vi "Configure Tx.vi"(0 "niUsrpRio Session":T1={"FPGA Interface"=refnum, "RIO Interface Number"=0, "Data Clock Rate"=0, "FPGA Data Clock Rate"=0, "Global Settings Register Bus"=refnum, "Radio 0 Settings Register Bus"=refnum, "Radio 1 Settings Register Bus"=refnum, "Radio Settings Bus Semaphore"=refnum, "DB Queues"=[], "Characterization Data Valid?"=FALSE, "EEPROM Header"={"Checksum"=0, "Product Code"=0, "Hardware Current Version"=0, "Hardware Oldest Compatible Version"=0, "EEPROM Map Current Version"=0, "EEPROM Map Oldest Compatible Version"=0, "User Password"="", "Pointer to Factory Header"=0, "Pointer to User Header"=0, "Recommended Interval"=0, "Number of Reserved Bytes"=9, "Number of Daughterboards"=0, "Daughterboard IDs"=[], "Daughterboard Serial Numbers"=[]}, "Device Data Header"={"Checksum"=0, "Number of Channels"=0, "Number of Gain Settings"=[], "Pointer to Characterization Data"=[], "Number of Reserved Bytes"=27, "Number of Frequencies"=[]}, "EEPROM Characterization Header"={"Checksum"=0, "Date"=timestamp(0 s since 1904-01-01), "Temperature"=0.0, "Misc. Info"="", "Pointer to Device Data Header"=0, "Number of Reserved Bytes"=28}, "Characterization Data"=[], "FPGA Current Version"=0, "FPGA Oldest Compatible Version"=0, "Fixed Logic Current Version"=0, "Fixed Logic Oldest Compatible Version"=0, "FPGA Radio Settings Bus Current Version"=0, "FPGA Radio Settings Bus Oldest Compatible Version"=0, "FPGA Board Config Current Version"=0, "FPGA Board Config Oldest Compatible Version"=0} {"FPGA Data Clock Rate" format="%#.3pHz"; "Data Clock Rate" format="%#.3pHz"; "Characterization Data"."Frequencies [Hz]" format="%#_6p"; "EEPROM Characterization Header"."Pointer to Device Data Header" format="%x"; "EEPROM Characterization Header"."Checksum" format="%x"; "Device Data Header"."Pointer to Characterization Data" format="%x"; "Device Data Header"."Checksum" format="%x"; "EEPROM Header"."Pointer to User Header" format="%x"; "EEPROM Header"."Pointer to Factory Header" format="%x"; "EEPROM Header"."Product Code" format="%x"; "EEPROM Header"."Checksum" format="%x"}, 5 "tx config":T11={"rf enable 0"=FALSE, "rf config 0"={"antenna"="TX1", "frequency"=2000000000.0, "lo frequency"=-1.0, "level"=0.0}, "rf enable 1"=FALSE, "rf config 1"={"antenna"="TX1", "frequency"=2000000000.0, "lo frequency"=-1.0, "level"=0.0}, "transfer mode"=enum."Finite", "sample rate"=10000000.0, "number of samples"=8192, "start trigger"=enum."Immediate", "tone frequency"=100000.0} {"tone frequency" format="%#.3pHz"; "sample rate" format="%#.3pS/s"; "rf config 0"."level" format="%#_gdBm"; "rf config 0"."lo frequency" format="%#.3pHz"; "rf config 0"."frequency" format="%#.3pHz"; "rf config 1"."level" format="%#_gdBm"; "rf config 1"."lo frequency" format="%#.3pHz"; "rf config 1"."frequency" format="%#.3pHz"}, 11 "error in":errorcluster, 12 "x":cdb[](array[numeric])) -> (4 "niUsrpRio Session (out)":T1 {"FPGA Data Clock Rate" format="%#.3pHz"; "Data Clock Rate" format="%#.3pHz"; "Characterization Data"."Frequencies [Hz]" format="%#_6p"; "EEPROM Characterization Header"."Pointer to Device Data Header" format="%x"; "EEPROM Characterization Header"."Checksum" format="%x"; "Device Data Header"."Pointer to Characterization Data" format="%x"; "Device Data Header"."Checksum" format="%x"; "EEPROM Header"."Pointer to User Header" format="%x"; "EEPROM Header"."Pointer to Factory Header" format="%x"; "EEPROM Header"."Product Code" format="%x"; "EEPROM Header"."Checksum" format="%x"}, 6 "tx.enabled channels":string[](array[string]), 8 "I":i16[](array[numeric]), 10 "Q":i16[](array[numeric]), 13 "tx.output waveform":waveform(dbl)[](graph), 14 "tx.coerced configurations":T12 {"coerced sample rates" format="%#.3pS/s"; "coerced levels" format="%#.3gdBm"; "coerced lo frequencies" format="%#.3pHz"; "coerced frequencies" format="%#.3pHz"}, 15 "error out":errorcluster)   [LabVIEW 2015]
uses:
  <instrlib>/niUsrpRio/Config/v1/Host/Public/niUsrpRio Session.ctl
  <instrlib>/_niInstr/Register Bus/v0/Host/Public/Register Bus Session.ctl
  <instrlib>/_niInstr/Register Bus/v0/Host/Private/Session Data.ctl
  <instrlib>/niUsrpRio/Config/v1/Host/Private/DB Queue Reference.ctl
  <instrlib>/niUsrpRio/Config/v1/Host/Private/Daughterboard Data.ctl
  <instrlib>/niUsrpRio/Config/v1/Host/Private/ATR state data.ctl
  <instrlib>/niUsrpRio/Config/v1/Host/Public/EEPROM Header.ctl
  <instrlib>/niUsrpRio/Config/v1/Host/Public/EEPROM Device Data Header.ctl
  <instrlib>/niUsrpRio/Config/v1/Host/Public/EEPROM Characterization Header.ctl
  <instrlib>/niUsrpRio/Config/v1/Host/Public/Characterization Data.ctl
  <instrlib>/niUsrpRio/Config/v1/Host/Public/IQ Imbalance.ctl
  Start Trigger.ctl
  Configure Signal (Level).vi
  PPS_Global_Var.vi
  <instrlib>/_niInstr/Register Bus/v0/Host/niInstr Register Bus v0 Host.lvlib
  <instrlib>/niUsrpRio/Config/v1/Host/niUsrpRio Config v1 Host.lvlib
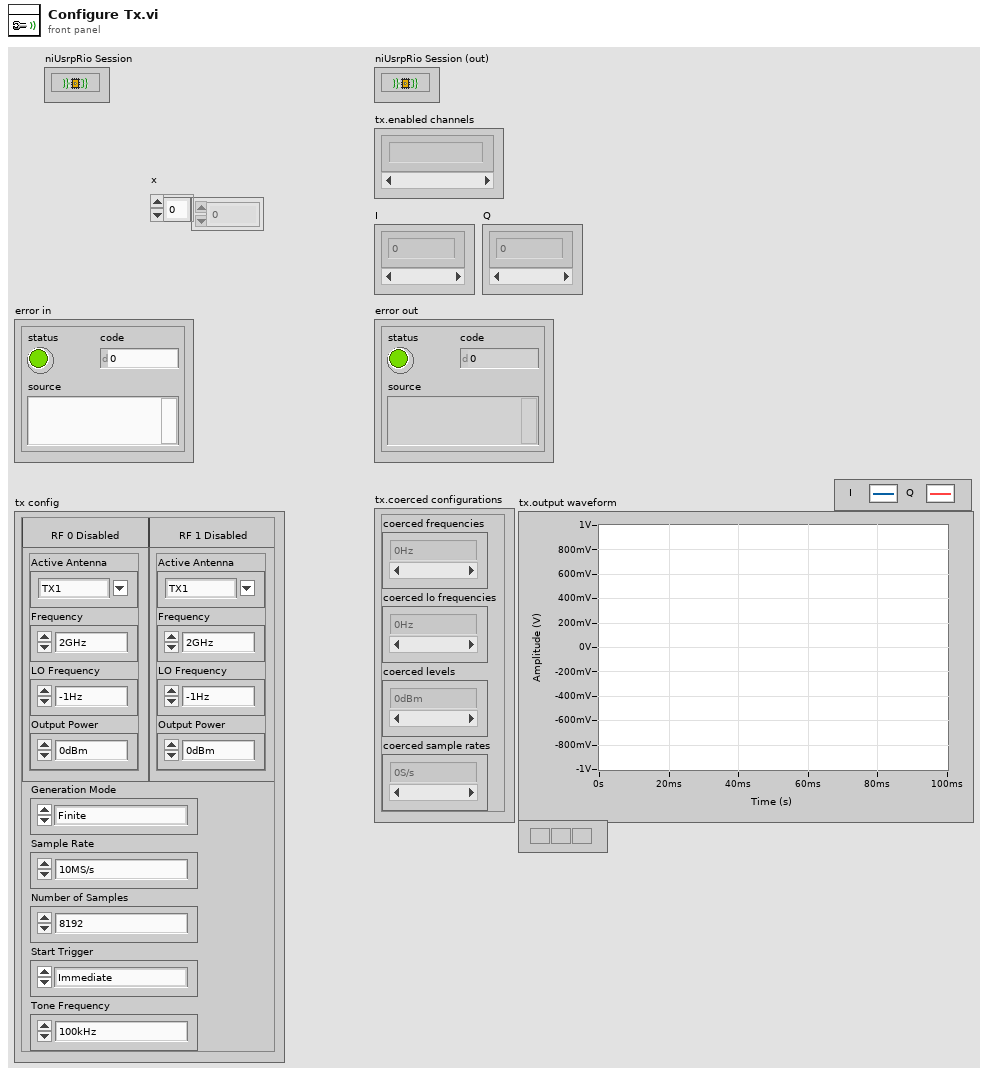
[diagram p1: front panel]
types:
  T1 = typedef "niUsrpRio Config v1 Host.lvlib/niUsrpRio Session.ctl" = cluster{"FPGA Interface":refnum<k20>, "RIO Interface Number":u32, "Data Clock Rate":u32, "FPGA Data Clock Rate":u32, "Global Settings Register Bus":T2, "Radio 0 Settings Register Bus":T2, "Radio 1 Settings Register Bus":T2, "Radio Settings Bus Semaphore":T3, "DB Queues":T4[], "Characterization Data Valid?":bool, "EEPROM Header":T5, "Device Data Header":T6, "EEPROM Characterization Header":T7, "Characterization Data":T8[], "FPGA Current Version":u32, "FPGA Oldest Compatible Version":u32, "Fixed Logic Current Version":u32, "Fixed Logic Oldest Compatible Version":u32, "FPGA Radio Settings Bus Current Version":u32, "FPGA Radio Settings Bus Oldest Compatible Version":u32, "FPGA Board Config Current Version":u32, "FPGA Board Config Oldest Compatible Version":u32}
  T2 = typedef "niInstr Register Bus v0 Host.lvlib/Register Bus Session.ctl" = refnum<queue>
  T3 = typedef "Semaphore RefNum" = refnum<k1>
  T4 = typedef "niUsrpRio Config v1 Host.lvlib/DB Queue Reference.ctl" = refnum<queue>
  T5 = typedef "niUsrpRio Config v1 Host.lvlib/EEPROM Header.ctl" = cluster{"Checksum":u32, "Product Code":u16, "Hardware Current Version":u16, "Hardware Oldest Compatible Version":u16, "EEPROM Map Current Version":u16, "EEPROM Map Oldest Compatible Version":u16, "User Password":string, "Pointer to Factory Header":u32, "Pointer to User Header":u32, "Recommended Interval":u16, "Number of Reserved Bytes":i32, "Number of Daughterboards":u8, "Daughterboard IDs":u16[], "Daughterboard Serial Numbers":string[]}
  T6 = typedef "niUsrpRio Config v1 Host.lvlib/EEPROM Device Data Header.ctl" = cluster{"Checksum":u32, "Number of Channels":u8, "Number of Gain Settings":u16[], "Pointer to Characterization Data":u32[], "Number of Reserved Bytes":i32, "Number of Frequencies":u16[]}
  T7 = typedef "niUsrpRio Config v1 Host.lvlib/EEPROM Characterization Header.ctl" = cluster{"Checksum":u32, "Date":timestamp, "Temperature":sgl, "Misc. Info":string, "Pointer to Device Data Header":u32, "Number of Reserved Bytes":i32}
  T8 = typedef "niUsrpRio Config v1 Host.lvlib/Characterization Data.ctl" = cluster{"Gains[dB]":dbl[], "Frequencies [Hz]":dbl[], "IQ Imbalance Table":T9[], "Measured Gains[dB]":dbl[][]}
  T9 = typedef "niUsrpRio Config v1 Host.lvlib/IQ Imbalance.ctl" = cluster{"Gain Imbalance [linear]":dbl, "Phase Imbalance [radians]":dbl, "Offset":cdb}
  T10 = typedef "Start Trigger.ctl" = enum8{"Software", "Digital Edge", "Rx Start Trigger", "Tx Start Trigger", "Immediate", "Future Time Event"}
  T11 = cluster{"rf enable 0":bool, "rf config 0":cluster{"antenna":string, "frequency":dbl, "lo frequency":dbl, "level":dbl}, "rf enable 1":bool, "rf config 1":cluster{"antenna":string, "frequency":dbl, "lo frequency":dbl, "level":dbl}, "transfer mode":enum16{"Finite", "Continuous"}, "sample rate":dbl, "number of samples":u32, "start trigger":T10, "tone frequency":dbl}
  T12 = cluster{"coerced frequencies":dbl[], "coerced lo frequencies":dbl[], "coerced levels":dbl[], "coerced sample rates":dbl[]}
  T13 = cluster{"antenna":string, "frequency":dbl, "lo frequency":dbl, "level":dbl}
  T14 = cluster{"rf enable 0":bool, "rf config 0":cluster{"antenna":string, "frequency":dbl, "lo frequency":dbl, "level":dbl}}
  T15 = cluster{"rf enable 1":bool, "rf config 1":cluster{"antenna":string, "frequency":dbl, "lo frequency":dbl, "level":dbl}}
  T16 = cluster{"rf enable 1":bool, "rf config 1":cluster{"antenna":string, "frequency":dbl, "lo frequency":dbl, "level":dbl}}[]
  T17 = cluster{"antenna":string, "frequency":dbl, "lo frequency":dbl, "level":dbl}[]
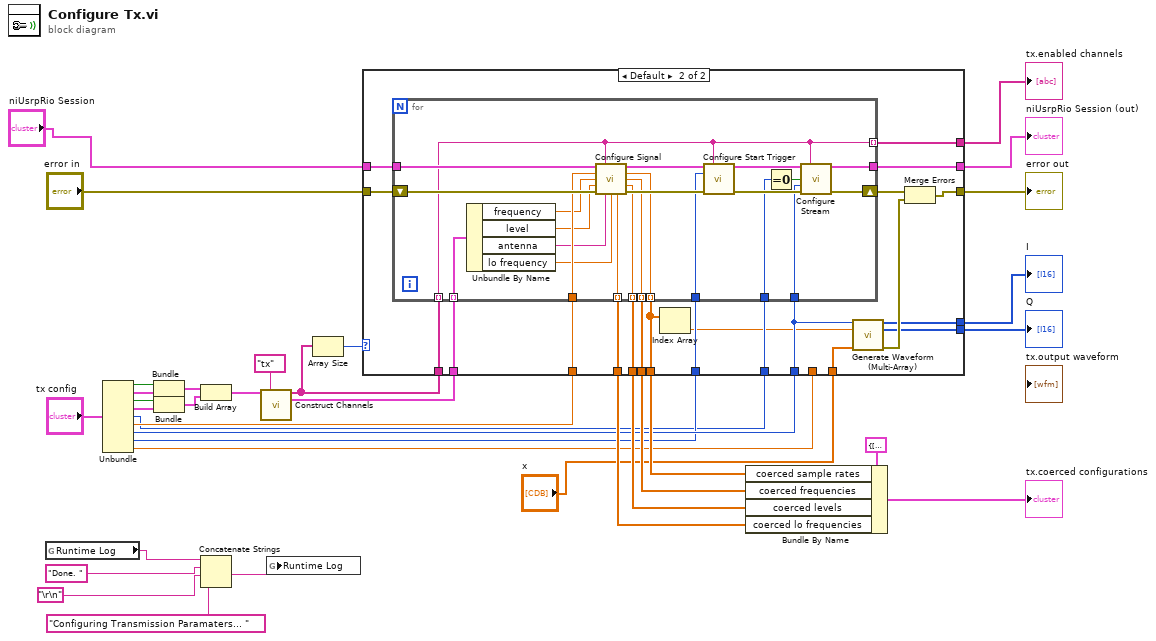
[diagram p0: block diagram]
diagram:
  n1 = global read "PPS_Global_Var.vi" "Runtime Log"() -> (w4:string)
  n2 = Unbundle("tx config") -> ("rf enable 0"=w23:bool, "rf config 0"=w22:T13, "rf enable 1"=w21:bool, "rf config 1"=w20:T13, "transfer mode"=w12:enum16{"Finite", "Continuous"}, "sample rate"=w19:dbl, "number of samples"=w14:u32, "start trigger"=w13:T10, "tone frequency"=w11:dbl)
  n3 = Bundle("rf enable 0"=w23, "rf config 0"=w22) -> (w31:T14)  [unwired: 1 in]
  n4 = Bundle("rf enable 1"=w21, "rf config 1"=w20) -> (w30:T15)  [unwired: 1 in]
  n5 = Build Array(w31, w30) -> (w28:T16)
  n6 = Concatenate Strings(w4, "Done. ", "\r\n", "Configuring Transmission Paramaters... ") -> (w5:string)
  n7 = call "Construct Channels.vi"("channel configurations"=w28, "scope"="tx") -> ("enabled channels"=w15:string[], "enabled channel configurations"=w29:T17)  [unwired: 12 in]
  n8 = global write "PPS_Global_Var.vi" "Runtime Log"(w5) -> ()
  n9 = Array Size(array=w15) -> (size(s)=w16:i32)
  n10 = case shown="Default" w16 {
    tunnel: [_ w41] -> w36
    tunnel: [_ w59] -> w35
    tunnel: [_ w58] -> w34
    tunnel: [_ w57] -> w33
    tunnel: w13 -> [_ w56]
    tunnel: w15 -> [_ w55]
    tunnel: w29 -> [_ w54]
    tunnel: [_ w53] -> w27
    tunnel: w19 -> [_ w47]
    tunnel: w12 -> [_ w52]
    tunnel: w14 -> [_ w46]
    tunnel: [w38 w51] -> w18
    tunnel: "error in" -> [w37 w50]
    tunnel: "niUsrpRio Session" -> [w38 w49]
    tunnel: [w37 w45] -> w32
    tunnel: w11 -> [_ _]
    tunnel: [_ w43] -> w10
    tunnel: [_ w42] -> w9
    tunnel: "x" -> [_ w39]
    frame 0 {
    }
    frame Default {
      n11 = for "channel configuration" {
        tunnel: [w76] -> w57 mode=indexing
        tunnel: w56 -> [w78]
        tunnel: w46 -> [w62]
        tunnel: w52 -> [w77]
        shift-right: [w61] -> w48
        shift-left: w50 -> [w82]
        tunnel: w47 -> [w81]
        tunnel: [w75] -> w58 mode=indexing
        tunnel: [w74] -> w59 mode=indexing
        tunnel: [w73] -> w41 mode=indexing
        tunnel: w54 -> [w72] mode=indexing
        tunnel: w55 -> [w69] mode=indexing
        tunnel: [w69] -> w53 mode=indexing
        tunnel: [w71] -> w51
        tunnel: w49 -> [w70]
        n12 = Unbundle By Name(w72) -> ("frequency"=w66:dbl, "level"=w63:dbl, "antenna"=w65:string, "lo frequency"=w64:dbl)
        n13 = call-poly "Configure Signal.vi"("niUsrpRio Session"=w70, "scope"=w69, "sample rate [S/s]"=w81, "frequency [Hz]"=w66, "level [dBm]"=w63, "error in"=w82, "Active Antenna"=w65, "LO frequency [Hz]"=w64) -> ("niUsrpRio Session (out)"=w68:T1, "coerced sample rate [S/s]"=w73:dbl, "coerced frequency [Hz]"=w74:dbl, "coerced level [dBm]"=w75:dbl, "coerced LO frequency [Hz]"=w76:dbl, "error out"=w80:errorcluster)  [unwired: 1 in, 1 out]
        n14 = call "Configure Start Trigger.vi"("niUsrpRio Session"=w68, "scope"=w69, "start trigger"=w78, "error in"=w80) -> ("niUsrpRio Session (out)"=w67:T1, "error out"=w79:errorcluster)  [unwired: 10 in]
        n15 = Equal To 0?(x=w77) -> (x = 0?=w60:bool)
        n16 = call "Configure Stream.vi"("niUsrpRio Session"=w67, "scope"=w69, "number of samples is finite"=w60, "number of samples"=w62, "error in"=w79) -> ("niUsrpRio Session (out)"=w71:T1, "error out"=w61:errorcluster)  [unwired: 9 in]
      }
      n17 = Index Array(array=w41) -> (element=w40:dbl)  [unwired: 1 in]
      n18 = call "Generate Waveform (Multi-Array).vi"("number of samples"=w46, "sample rate"=w40, "x"=w39) -> ("I"=w43:i16[], "Q"=w42:i16[], "error out"=w44:errorcluster)  [unwired: 10 in]
      n19 = Merge Errors(w48, w44) -> (w45:errorcluster)
    }
  }
  "niUsrpRio Session (out)" <- w18
  "error out" <- w32
  "tx.enabled channels" <- w27
  "I" <- w10
  "Q" <- w9
  n20 = Bundle By Name(cluster=T12 {"coerced frequencies"=[], "coerced lo frequencies"=[], "coerced levels"=[], "coerced sample rates"=[]} ("coerced configurations"), "coerced sample rates"=w36, "coerced frequencies"=w35, "coerced levels"=w34, "coerced lo frequencies"=w33) -> (→"tx.coerced configurations":T12)
